vi "Align Front Panel.vi"(8 "error in (no error)":errorcluster, 11 "VI Refnum In (Calling VI)":refnum<vi>) -> (0 "error out":errorcluster, 3 "VI Refnum out":refnum<vi>)   [LabVIEW 2013, in "DCAF UI Elements.lvlib"]
uses:
  Controls/DCAF UI Elements.lvlib
  <vilib>/Utility/miscctls.llb/LVRectTypeDef.ctl
  <vilib>/Utility/miscctls.llb/LVPointTypeDef.ctl
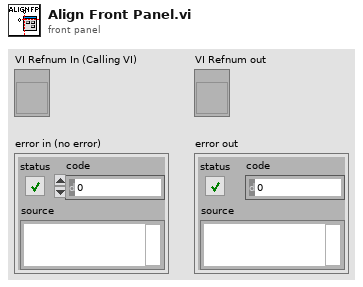
[diagram p1: front panel]
types:
  T1 = typedef "LVPointTypeDef.ctl" = cluster{"Horizontal":i16, "Vertical":i16}
  T2 = typedef "LVRectTypeDef.ctl" = cluster{"Left":i16, "Top":i16, "Right":i16, "Bottom":i16}
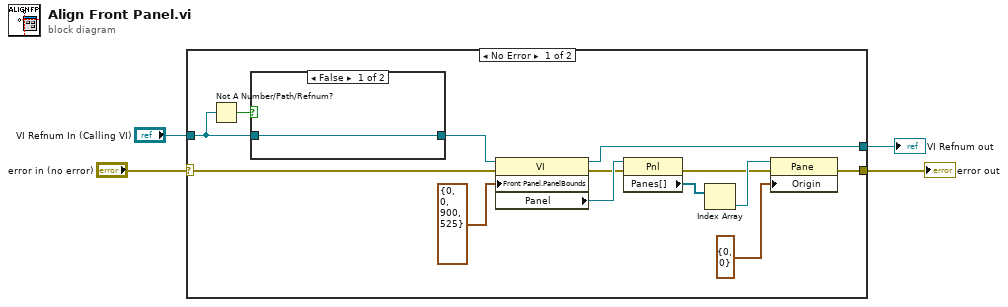
[diagram p0: block diagram]
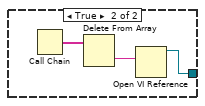
[diagram p2: hidden frame]
diagram:
  n1 = case shown="No Error" "error in (no error)" {
    selector: "error in (no error)" -> [w8 w22]
    tunnel: "VI Refnum In (Calling VI)" -> [w6 w23]
    tunnel: [w10 w23] -> w3
    tunnel: [w9 w22] -> w2
    frame No Error {
      n2 = Not A Number/Path/Refnum?(number/path/refnum=w6) -> (NaN/Path/Refnum?=w7:bool)
      n3 = case shown="False" w7 {
        tunnel: w6 -> [w18 _]
        tunnel: [w18 w19] -> w5
        frame False {
        }
        frame True {
          n4 = Call Chain() -> (call chain=w21:string[])
          n5 = Delete From Array(array=w21) -> (deleted portion=w20:string)  [unwired: 2 in, 1 out]
          n6 = Open VI Reference(vi path=w20) -> (vi reference=w19:refnum<vi>)  [unwired: 5 in, 1 out]
        }
      }
      n7 = property class="VI"(reference=w5, error in=w8, "Front Panel.PanelBounds"=T2 {"Left"=0, "Top"=0, "Right"=900, "Bottom"=525} ("Front Panel Window:Panel Bounds")) -> (reference out=w10:refnum<vi>, error out=w12:errorcluster, "Panel"=w16:refnum<vi>)
      n8 = property class="Pnl"(reference=w16, error in=w12) -> (error out=w11:errorcluster, "Panes[]"=w15:refnum<vi>[])  [unwired: 1 out]
      n9 = Index Array(array=w15) -> (element=w14:refnum<vi>)  [unwired: 1 in]
      n10 = property class="Pane"(reference=w14, error in=w11, "Origin"=T1 {"Horizontal"=0, "Vertical"=0}) -> (error out=w9:errorcluster)  [unwired: 1 out]
    }
    frame Error {
    }
  }
  "VI Refnum out" <- w3
  "error out" <- w2
